vi "AI Timestamp Accuracy.vi"() -> ()   [LabVIEW 2020]
uses:
  <vilib>/DAQmx/write.llb/DAQmx Write (Digital Bool 1Line 1Point).vi
  <vilib>/DAQmx/read.llb/DAQmx Read (Analog Wfm 1Chan NSamp).vi
  33bc07a8-6ad9-4bf6-9483-3c817cfe2bbf.vi
  <vilib>/DAQmx/create/channels.llb/DAQmx Create Channel (AI-Voltage-Basic).vi
  <vilib>/DAQmx/configure/timing.llb/DAQmx Timing (Sample Clock).vi
  <vilib>/DAQmx/create/channels.llb/DAQmx Create Channel (DO-Digital Output).vi
  <vilib>/DAQmx/miscellaneous.llb/DAQmx Fill In Error Info.vi
panel:
  out "Iteration":i32
  out "finished":bool
  out "Graph":dbl[](graph)
  out "Array 3":dbl[](array[numeric]) format="%.6f"
  out "Array 2":dbl[](array[numeric]) format="%.6f"
  out "Array":dbl[](array[numeric]) format="%.6f"
  out "Graph":waveform(dbl)(graph)
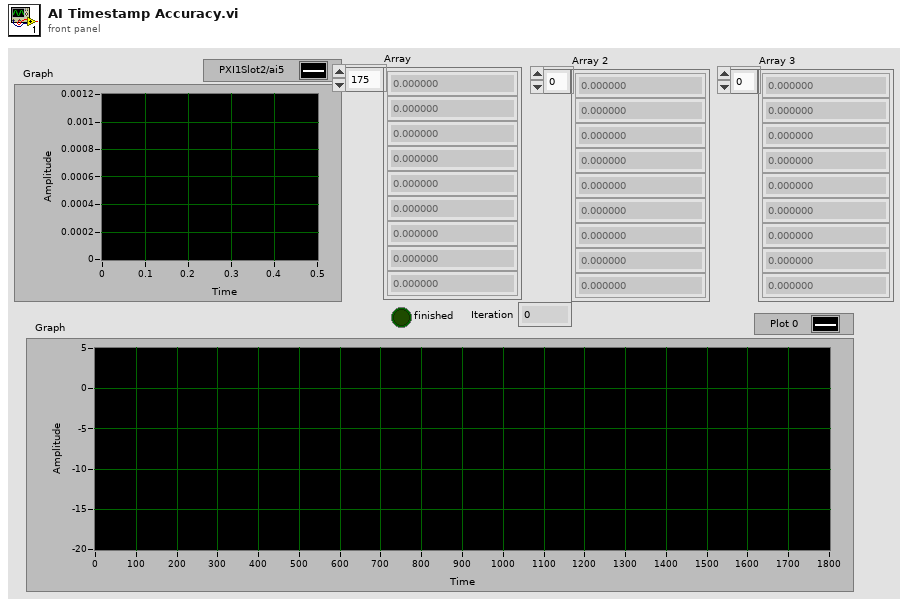
[diagram p1: front panel]
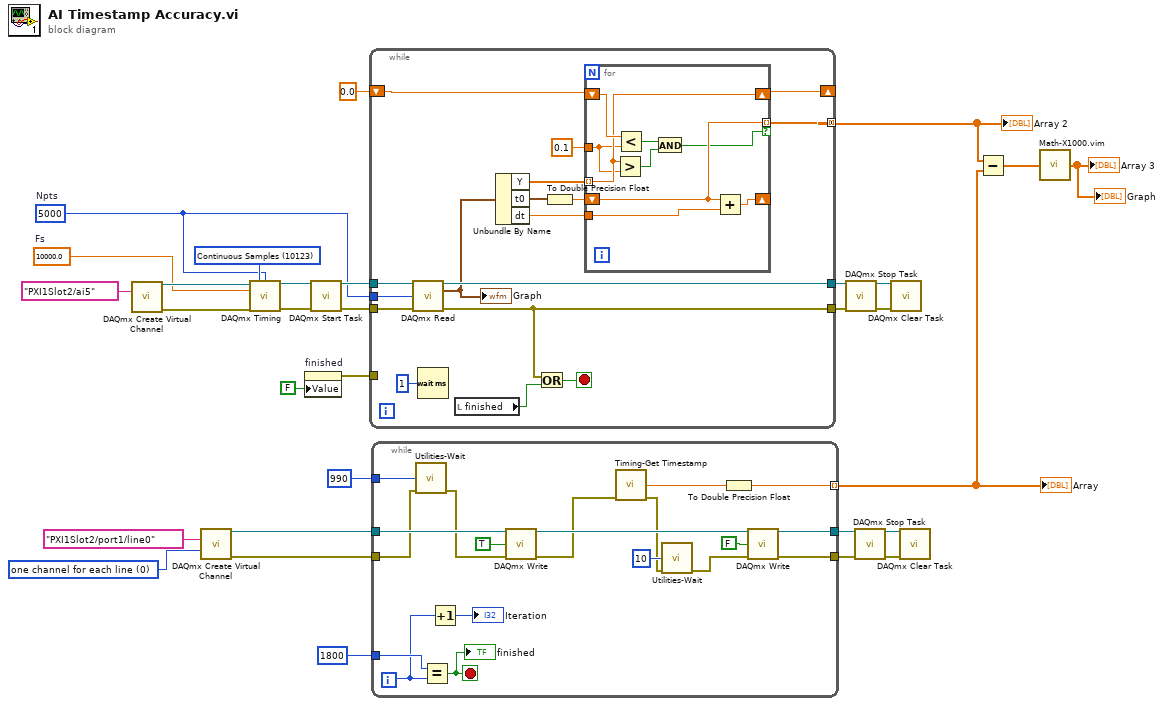
[diagram p0: block diagram]
diagram:
  w17 = 0 items=["one channel for each line", "one channel for all lines"] ("line grouping")
  w11 = 10000.0  # Fs
  w12 = 5000  # Npts
  w29 = 10123 items=["Finite Samples"=10178, "Continuous Samples"=10123, "Hardware Timed Single Point"=12522] ("sample mode")
  n1 = call-poly <vilib>:"DAQmx Create Virtual Channel.vi"("physical channels"=tag "PXI1Slot2/ai5") -> ("task out"=w31:refnum<k21>, "error out"=w30:errorcluster)  [unwired: 13 in]
  n2 = call-poly <vilib>:"DAQmx Create Virtual Channel.vi"("lines"=tag "PXI1Slot2/port1/line0", "line grouping"=w17) -> ("task out"=w18:refnum<k21>, "error out"=w4:errorcluster)  [unwired: 12 in]
  n3 = call-poly <vilib>:"DAQmx Timing.vi"("task/channels in"=w31, "sample mode"=w29, "samples per channel"=w12, "rate"=w11, "error in"=w30) -> ("task out"=w21:refnum<k21>, "error out"=w20:errorcluster)  [unwired: 9 in]
  n4 = property on="finished" class="Bool (strict)"("Value"=FALSE ("finished")) -> (error out=w2:errorcluster)  [unwired: 2 in, 1 out]
  n5 = call <vilib>:"DAQmx Start Task.vi"("task/channels in"=w21, "error in"=w20) -> ("task out"=w27:refnum<k21>, "error out"=w28:errorcluster)  [unwired: 12 in]
  n6 = while {
    tunnel: w28 -> [w46]
    tunnel: w27 -> [w47]
    tunnel: [w45] -> w26
    tunnel: [w43] -> w25
    tunnel: w12 -> [w44]
    shift-right: [w40] -> _
    shift-left: 0.0 -> [w41]
    tunnel: [w34] -> w9 mode=concatenating
    tunnel: w2 -> [_]
    stop <- w33 stop-if-true
    n7 = call-poly <vilib>:"DAQmx Read.vi"("task/channels in"=w47, "number of samples per channel"=w44, "error in"=w46) -> ("task out"=w45:refnum<k21>, "data"=w42:waveform(dbl), "error out"=w43:errorcluster)  [unwired: 10 in]
    "Graph" <- w42
    n8 = Wait (ms)(milliseconds to wait=u32 1) -> ()  [unwired: 1 out]
    n9 = local read "finished"() -> (w32:bool)
    n10 = Unbundle By Name(w42) -> ("Y"=w39:dbl[], "t0"=w37:timestamp, "dt"=w35:dbl)
    n11 = Or(x=w43, y=w32) -> (x .or. y?=w33:bool)
    n12 = To Double Precision Float(number=w37) -> (double precision float=w36:dbl)
    n13 = for {
      tunnel: w39 -> [w56] mode=indexing
      shift-right: [w56] -> w40
      shift-left: w41 -> [w57]
      tunnel: 0.1 -> [w55]
      tunnel: w35 -> [w51]
      shift-right: [w52] -> _
      shift-left: w36 -> [w50]
      tunnel: [w50] -> w34 mode=indexing if=w49
      n14 = Greater?(x=w56, y=w55) -> (0:w53:bool)
      n15 = Less?(x=w57, y=w55) -> (x < y?=w54:bool)
      n16 = And(x=w54, y=w53) -> (x .and. y?=w49:bool)
      n17 = Add(x=w50, y=w51) -> (x+y=w52:dbl)
    }
  }
  "Array 2" <- w9
  n18 = while {
    tunnel: w18 -> [w76]
    tunnel: [w70] -> w14
    tunnel: [w69] -> w13
    tunnel: [w68] -> w8 mode=indexing
    tunnel: 1800 ("x") -> [w67]
    tunnel: u32 990 ("milliseconds to wait") -> [w65]
    tunnel: w4 -> [w64]
    i -> [w58]
    stop <- w60 stop-if-true
    n19 = call "Utilities-Wait.vi"("milliseconds to wait"=w65, "error in (no error)"=w64) -> ("error out"=w63:errorcluster)  [unwired: 13 in]
    n20 = Equal?(x=w67, y=w58) -> (x = y?=w60:bool)
    "finished" <- w60
    n21 = Increment(x=w58) -> (x+1=→"Iteration":i32)
    n22 = call-poly <vilib>:"DAQmx Write.vi"("task/channels in"=w76, "data"=TRUE, "error in"=w63) -> ("task out"=w73:refnum<k21>, "error out"=w62:errorcluster)  [unwired: 10 in, 1 out]
    n23 = call "Timing-Get Timestamp.vi"("error in (no error)"=w62) -> ("double precision float"=w66:dbl, "error out"=w61:errorcluster)  [unwired: 13 in]
    n24 = call "Utilities-Wait.vi"("milliseconds to wait"=u32 10, "error in (no error)"=w61) -> ("error out"=w72:errorcluster)  [unwired: 13 in]
    n25 = To Double Precision Float(number=w66) -> (double precision float=w68:dbl)
    n26 = call-poly <vilib>:"DAQmx Write.vi"("task/channels in"=w73, "data"=FALSE, "error in"=w72) -> ("task out"=w70:refnum<k21>, "error out"=w69:errorcluster)  [unwired: 10 in, 1 out]
  }
  "Array" <- w8
  n27 = call <vilib>:"DAQmx Stop Task.vi"("task/channels in"=w26, "error in"=w25) -> ("task out"=w24:refnum<k21>, "error out"=w23:errorcluster)  [unwired: 12 in]
  n28 = call <vilib>:"DAQmx Stop Task.vi"("task/channels in"=w14, "error in"=w13) -> ("task out"=w16:refnum<k21>, "error out"=w15:errorcluster)  [unwired: 12 in]
  n29 = call <vilib>:"DAQmx Clear Task.vi"("task in"=w24, "error in"=w23) -> ()  [unwired: 13 in, 1 out]
  n30 = call <vilib>:"DAQmx Clear Task.vi"("task in"=w16, "error in"=w15) -> ()  [unwired: 13 in, 1 out]
  n31 = Subtract(x=w9, y=w8) -> (x-y=w7:dbl[])
  n32 = call "Math-X1000.vim"("X"=w7) -> ("1000X"=→"Array 3" →"Graph":dbl[])
